vi "Table Select Section Copy to 1D Array.vi"(11 "Table Ref In":refnum<vi>) -> (1 "Copied Value":string[](array[string]), 3 "Table Ref Out":refnum<vi>)   [LabVIEW 2024]
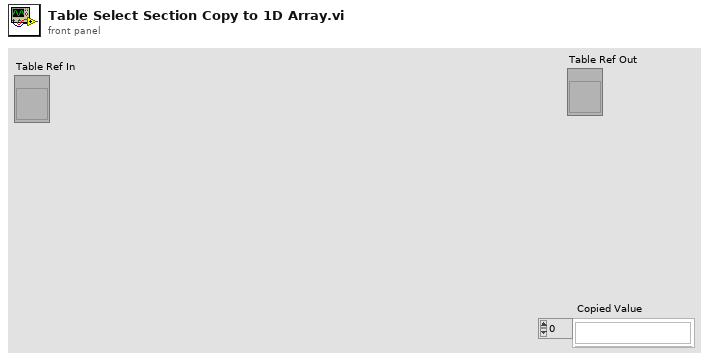
[diagram p1: front panel]
types:
  T1 = typedef "LVRowAndColumnTypeDef.ctl" = cluster{"Row":i32, "Column":i32}
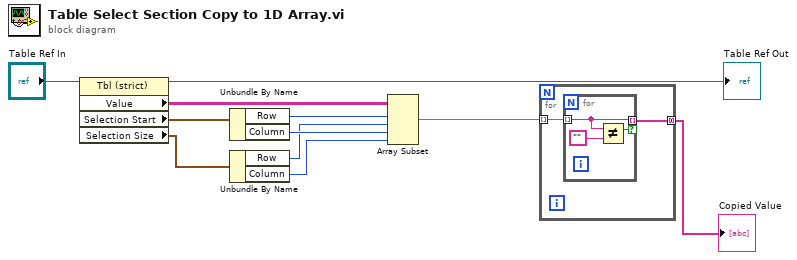
[diagram p0: block diagram]
diagram:
  n1 = property class="Tbl (strict)"(reference="Table Ref In") -> (reference out=→"Table Ref Out":refnum<vi>, "Value"=w2:string[][], "Selection Start"=w9:T1, "Selection Size"=w7:T1)  [unwired: 1 in, 1 out]
  n2 = Unbundle By Name(w9) -> ("Row"=w1:i32, "Column"=w8:i32)
  n3 = Unbundle By Name(w7) -> ("Row"=w6:i32, "Column"=w5:i32)
  n4 = Array Subset(array=w2, index (row)=w1, length (row)=w6, index (col)=w8, length (col)=w5) -> (w4:string[][])
  n5 = for {
    tunnel: w4 -> [w13] mode=indexing
    tunnel: [w12] -> w3 mode=concatenating
    n6 = for {
      tunnel: w13 -> [w15] mode=indexing
      tunnel: [w15] -> w12 mode=indexing if=w14
      n7 = Not Equal?(x=w15, y="") -> (x != y?=w14:bool)
    }
  }
  "Copied Value" <- w3
